vi "Combination to channel enable_2.vi"(1 "Channel":u16=9764, 2 "Channel Combination":u32=9764) -> (0 "Enable":bool)   [LabVIEW 2012]
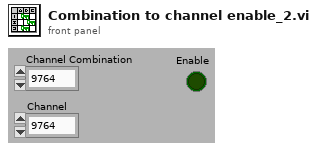
[diagram p1: front panel]
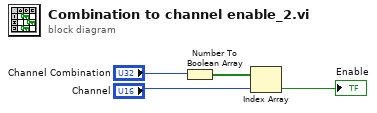
[diagram p0: block diagram]
diagram:
  n1 = Number To Boolean Array(number="Channel Combination") -> (Boolean array=w4:bool[])
  n2 = Index Array(array=w4, index="Channel") -> (element=→"Enable":bool)
